vi "Actuation_VideoTest.vi"() -> ()   [LabVIEW 2024]
panel:
  out "error out":errorcluster
  in  "go":bool
  in  "TempPoint":i32=-66
  in  "TempCycleNo":i32=1
  in  "TopFolderPath":path=path "E:/LTM Tests"
  in  "TopFolderPrefix":string="WednesDay"
  out "Actuation Logging":bool
  out "Heater Logging":bool
  in  "Actuation Post-Log(s)":dbl=1.0 format="%#_13g"
  in  "Actuation Pre-Log (s)":dbl=1.0 format="%#_13g"
  in  "COM Port":i32=21 min=1 max=63 step=1
  out "Camera":string="USB Camera"
  in  "Path to Actuation Script":path=path "C:/Users/dpl/OneDrive - Aberystwyth University/Documents/GitHub/Enfys-OBEGSE/ob_egse/egse.py"
  in  "FFMPEG exe":path=path "C:/Program Files/FFMpeg/bin/ffmpeg.exe"
  in  "PSU_Monitor":waveform(dbl)[](array[waveform])=[{"t0"=timestamp(3820238929.2708097 s since 1904-01-01), "dt"=1.0, "Y"=[-0.003], "attributes"=variant("NI_ChannelName"=variant(string "Board_Voltage_0"))}, {"t0"=timestamp(3820238929.279827 s since 1904-01-01), "dt"=1.0, "Y"=[-0.01], "attributes"=variant("NI_ChannelName"=variant(string "Board_Voltage_0"))}]
  in  "Heater Monitor":waveform(dbl)[](array[waveform])
  in  "TLUP_Temperatures":waveform(dbl)[](array[waveform])=[{"t0"=timestamp(3820239419.3012686 s since 1904-01-01), "dt"=1.0, "Y"=[-999.0], "attributes"=variant("NI_ChannelName"=variant(string "TLUP_0"))}, {"t0"=timestamp(3820239419.3012686 s since 1904-01-01), "dt"=1.0, "Y"=[-999.0], "attributes"=variant("NI_ChannelName"=variant(string "TLUP_1"))}, {"t0"=timestamp(3820239419.3012686 s since 1904-01-01), "dt"=1.0, "Y"=[-999.0], "attributes"=variant("NI_ChannelName"=variant(string "TLUP_2"))}, {"t0"=timestamp(3820239419.3012686 s since 1904-01-01), "dt"=1.0, "Y"=[-999.0], "attributes"=variant("NI_ChannelName"=variant(string "TLUP_3"))}, {"t0"=timestamp(3820239419.3012686 s since 1904-01-01), "dt"=1.0, "Y"=[nan], "attributes"=variant("NI_ChannelName"=variant(string "TLUP_4"))}, {"t0"=timestamp(3820239419.3012686 s since 1904-01-01), "dt"=1.0, "Y"=[nan], "attributes"=variant("NI_ChannelName"=variant(string "TLUP_5"))}, {"t0"=timestamp(3820239419.3012686 s since 1904-01-01), "dt"=1.0, "Y"=[nan], "attributes"=variant("NI_ChannelName"=variant(string "TLUP_6"))}, {"t0"=timestamp(3820239419.3012686 s since 1904-01-01), "dt"=1.0, "Y"=[nan], "attributes"=variant("NI_ChannelName"=variant(string "TLUP_7"))}]
  in  "TVC_Temperatures":waveform(dbl)[](array[waveform])=[{"t0"=timestamp(3820239418.4664574 s since 1904-01-01), "dt"=1.0, "Y"=[nan], "attributes"=variant("NI_ChannelName"=variant(string "3A"))}, {"t0"=timestamp(3820239418.4664574 s since 1904-01-01), "dt"=1.0, "Y"=[nan], "attributes"=variant("NI_ChannelName"=variant(string "3B"))}, {"t0"=timestamp(3820239418.4664574 s since 1904-01-01), "dt"=1.0, "Y"=[nan], "attributes"=variant("NI_ChannelName"=variant(string "3C"))}, {"t0"=timestamp(3820239418.4664574 s since 1904-01-01), "dt"=1.0, "Y"=[nan], "attributes"=variant("NI_ChannelName"=variant(string "3D"))}, {"t0"=timestamp(3820239418.4664574 s since 1904-01-01), "dt"=1.0, "Y"=[nan], "attributes"=variant("NI_ChannelName"=variant(string "4A"))}, {"t0"=timestamp(3820239418.4664574 s since 1904-01-01), "dt"=1.0, "Y"=[nan], "attributes"=variant("NI_ChannelName"=variant(string "4B"))}, {"t0"=timestamp(3820239418.4664574 s since 1904-01-01), "dt"=1.0, "Y"=[23.129], "attributes"=variant("NI_ChannelName"=variant(string "4C"))}, {"t0"=timestamp(3820239418.4664574 s since 1904-01-01), "dt"=1.0, "Y"=[nan], "attributes"=variant("NI_ChannelName"=variant(string "4D"))}, {"t0"=timestamp(3820239418.4664574 s since 1904-01-01), "dt"=1.0, "Y"=[15.0], "attributes"=variant("NI_ChannelName"=variant(string "Target"))}]
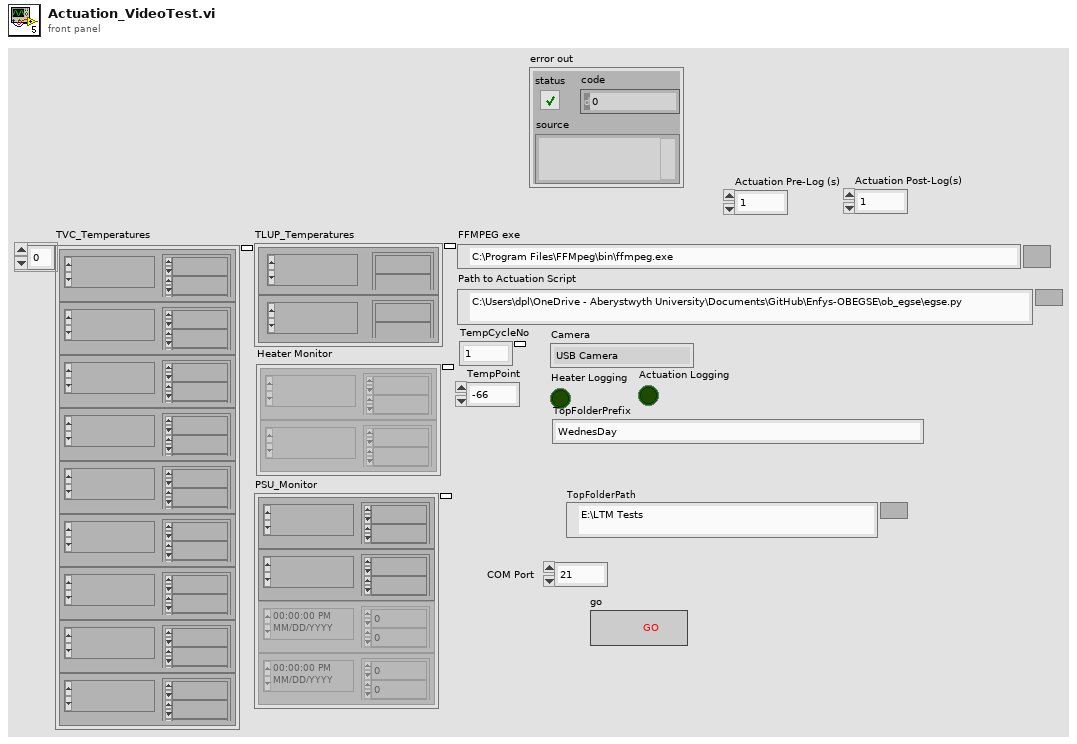
[diagram p1: front panel]
types:
  T1 = typedef "FFMpegRef.ctl" = cluster{"FFMpegRef":refnum<k24>, "StdOutRef":refnum<k24>, "DiagRef":refnum<k24>}
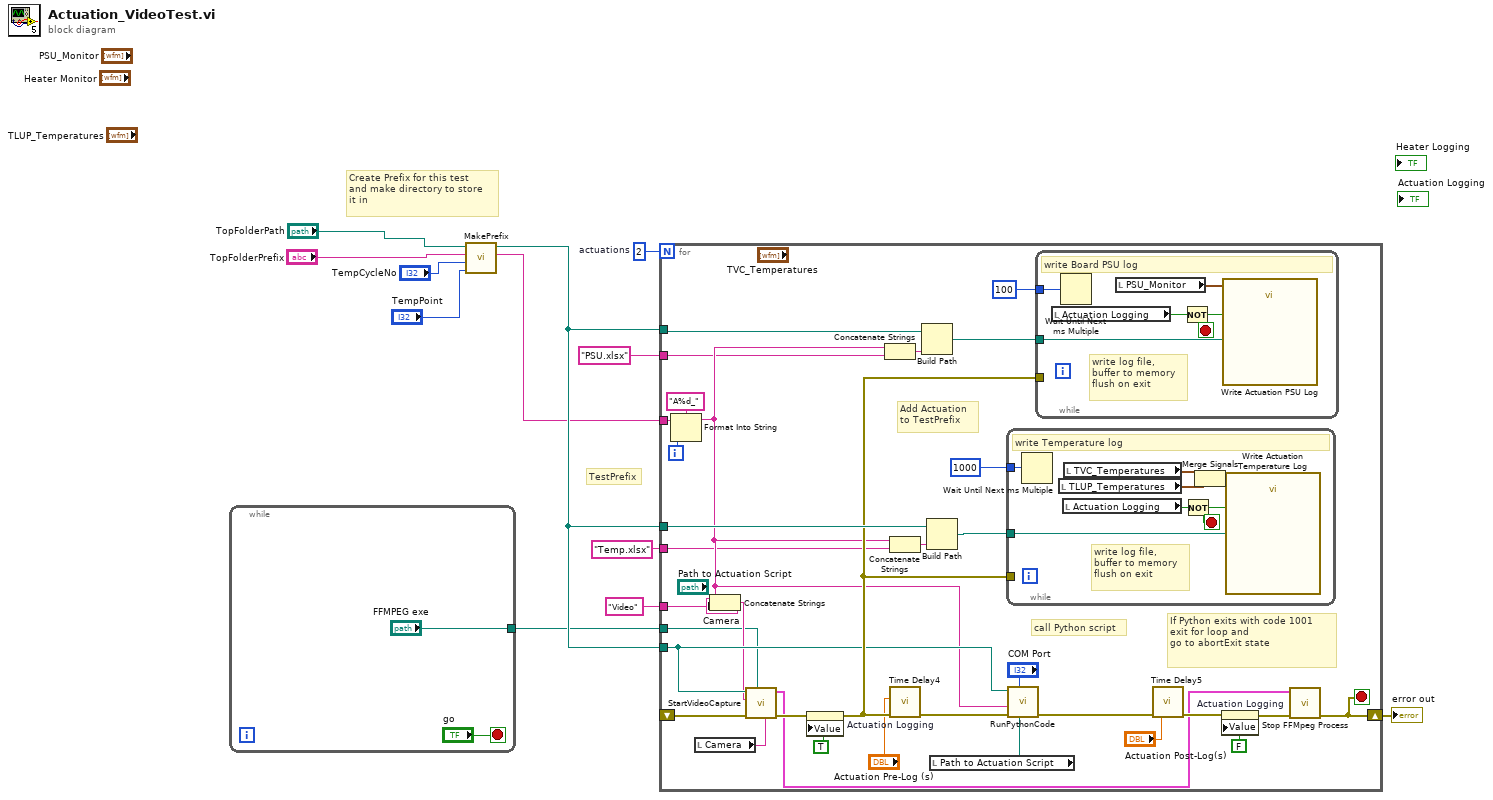
[diagram p0: block diagram]
diagram:
  w12 = 2  # actuations
  # "Create Prefix for this test\nand make directory to store \nit in"
  # "TestPrefix"
  n1 = while {
    tunnel: ["FFMPEG exe"] -> w2
    stop <- "go" stop-if-true
  }
  n2 = call "MakePrefix.vi"("TempPoint"="TempPoint", "TempCycleNo"="TempCycleNo", "FolderPrefix"="TopFolderPrefix", "TopFolderPath"="TopFolderPath") -> ("Prefix"=w6:string, "TestFolderPath"=w7:path)  [unwired: 6 in]
  n3 = for {
    N: w12 -> [_]
    shift-right: [w15] -> w1
    shift-left: _ -> [w29]
    tunnel: w6 -> [w27]
    tunnel: w7 -> [w43]
    tunnel: w7 -> [w36]
    tunnel: w7 -> [w31]
    tunnel: "Video" ("string") -> [w24]
    tunnel: "Temp.xlsx" ("string") -> [w23]
    tunnel: "PSU.xlsx" ("string") -> [w22]
    tunnel: w2 -> [w18]
    i -> [w45]
    stop <- w15 stop-if-true
    # "Add Actuation\nto TestPrefix"
    # "If Python exits with code 1001\nexit for loop and \ngo to abortExit state"
    # "call Python script"
    n4 = Format Into String(format string="A%d_", initial string=w27, w45) -> (resulting string=w25:string)  [unwired: 1 in, 1 out]
    n5 = local read "Camera"() -> (w28:string)
    n6 = Concatenate Strings(w25, w24) -> (w21:string)
    n7 = call "StartVideoCapture.vi"("Output Directory"=w31, "SaveFile"=w21, "error in (no error)"=w29, "Path to FFMPEG"=w18, "Video Camera"=w28) -> ("FFMpegProcess"=w17:T1, "error out"=w30:errorcluster)  [unwired: 4 in]
    n8 = property on="Actuation Logging" class="Bool (strict)"(error in=w30, "Value"=TRUE ("Actuation Logging")) -> (error out=w35:errorcluster)  [unwired: 1 in, 1 out]
    n9 = Concatenate Strings(w25, w22) -> (w41:string)
    n10 = Concatenate Strings(w25, w23) -> (w44:string)
    n11 = call "Time Delay4"("error in (no error)"=w35, "Delay Time (s)"="Actuation Pre-Log (s)") -> ("error out"=w39:errorcluster)  [unwired: 9 in]
    n12 = Build Path(base path=w36, name or relative path=w41) -> (appended path=w40:path)
    n13 = Build Path(base path=w43, name or relative path=w44) -> (appended path=w42:path)
    n14 = local read "Path to Actuation Script"() -> (w32:path)
    n15 = while {
      tunnel: w42 -> [w55]
      tunnel: w35 -> [_]
      tunnel: u32 1000 ("millisecond multiple") -> [w49]
      stop <- w53 stop-if-true
      # "write log file, \nbuffer to memory\nflush on exit"
      # "write Temperature log"
      n16 = Wait Until Next ms Multiple(millisecond multiple=w49) -> ()  [unwired: 1 out]
      n17 = local read "TLUP_Temperatures"() -> (w50:waveform(dbl)[])
      n18 = local read "Actuation Logging"() -> (w52:bool)
      n19 = local read "TVC_Temperatures"() -> (w51:waveform(dbl)[])
      n20 = Not(x=w52) -> (.not. x?=w53:bool)
      n21 = Merge Signals(w51, w50) -> (w54:dynamicdata)
      n22 = call "Write Actuation Temperature Log"("Signals"=w54, "Flush? (T)"=w53, "Filename"=w55) -> ()  [unwired: 14 in, 3 out]
    }
    n23 = call "RunPythonCode.vi"("Path to Actuation Script"=w32, "COM Port"="COM Port", "error in (no error)"=w39, "TestPrefix"=w25, "Output base directory"=w31) -> ("error out"=w38:errorcluster)  [unwired: 5 in, 1 out]
    n24 = while {
      tunnel: w40 -> [w59]
      tunnel: w35 -> [_]
      tunnel: u32 100 ("millisecond multiple") -> [w56]
      stop <- w57 stop-if-true
      # "write log file, \nbuffer to memory\nflush on exit"
      # "write Board PSU log"
      n25 = local read "Actuation Logging"() -> (w58:bool)
      n26 = Wait Until Next ms Multiple(millisecond multiple=w56) -> ()  [unwired: 1 out]
      n27 = local read "PSU_Monitor"() -> (w60:waveform(dbl)[])
      n28 = Not(x=w58) -> (.not. x?=w57:bool)
      n29 = call "Write Actuation PSU Log"("Signals"=w60, "Flush? (T)"=w57, "Filename"=w59) -> ()  [unwired: 14 in, 3 out]
    }
    n30 = call "Time Delay5"("error in (no error)"=w38, "Delay Time (s)"="Actuation Post-Log(s)") -> ("error out"=w37:errorcluster)  [unwired: 9 in]
    n31 = property on="Actuation Logging" class="Bool (strict)"(error in=w37, "Value"=FALSE ("Actuation Logging")) -> (error out=w26:errorcluster)  [unwired: 1 in, 1 out]
    n32 = call "Stop FFMpeg Process.vi"("error in (no error)"=w26, "FFMpegProcess"=w17) -> ("error out"=w15:errorcluster)  [unwired: 9 in]
  }
  "error out" <- w1
